vi "VGA_Loop.vi"   [LabVIEW 2019, in "VGA.lvlib"]
doc: "Contains the Loop to handle the VGA Output. It constantly outputs the FrameBuffer Memory. Update the FrameBuffer or change Initial-value of the Memory to display something."
uses:
  VGA.lvlib
  data.ctl
  <vilib>/Platform/TimedLoop/XDataNode/timing_clust.ctl
  <vilib>/Platform/TimedLoop/XDataNode/nitl_modes.ctl
  <vilib>/Platform/TimedLoop/XDataNode/wakeup.ctl
  <vilib>/rvi/Emulation/niFpgaSctlEmulationGetInTimedLoop.vi
  <vilib>/rvi/Emulation/niFpgaEmulationReportErrorSimple.vi
  <vilib>/rvi/Emulation/niFpgaGetClockAttributes.vi
  <vilib>/rvi/Emulation/niFpgaCriticalErrorInLSC.vi
  <vilib>/rvi/eio/common/nirviEmuTemplateMethod_errors.vi
  <vilib>/platform/TimedLoop/XDataNode/XDataNode.xnode
  <vilib>/eio/EIONode/EIONode.xnode
  <vilib>/Platform/TimedLoop/XDataNode/XDNodeRunTimeDep.lvlib
types:
  T1 = typedef "VGA.lvlib/data.ctl" = cluster{"x_frontporch":u8, "x_syncpulse":u8, "x_backporch":u8, "y_frontporch":u8, "y_syncpulse":u8, "y_backporch":u8, "DrawPixel?":bool, "x_tickcount":u16, "y_tickcount":u16, "x_Index":i16, "y_Index":i16}
  T2 = typedef "XDNodeRunTimeDep.lvlib/timing_clust.ctl" = cluster{"Expected End [f-1]":u64, "Actual End [f-1]":u64, "Finished Late? [f-1]":bool, "Expected End [i-1]":u64, "Actual End [i-1]":u64, "Finished Late? [i-1]":bool, "Expected Start [i]":u64, "Actual Start [i]":u64, "Expected Start [f]":u64, "Actual Start [f]":u64, "Source Name":string, "Structure Name":string, "Period":i64, "Deadline":i64, "Offset":i64, "Start":i64, "Priority":i32, "Timeout":i32, "Mode":T3, "Wakeup Reason":T4, "Error":errorcluster, "Source Type":string, "Secondary Source Type":string, "Global End Time":u64, "Global Start Time":u64, "Frame Duration":u64, "Iteration Duration":u64, "Assigned CPU":i32, "I/O Scan Engine Mode":u32}
  T3 = typedef "XDNodeRunTimeDep.lvlib/nitl_modes.ctl" = enum32{"No Change", "Process missed periods, maintain original phase", "Discard missed periods, maintain original phase", "Process missed periods, ignore original phase", "Discard missed periods, ignore original phase"}
  T4 = typedef "XDNodeRunTimeDep.lvlib/wakeup.ctl" = enum32{"Normal", "Aborted", "Asynchronous wakeup", "Timing source error", "Timed loop error", "Timeout"}
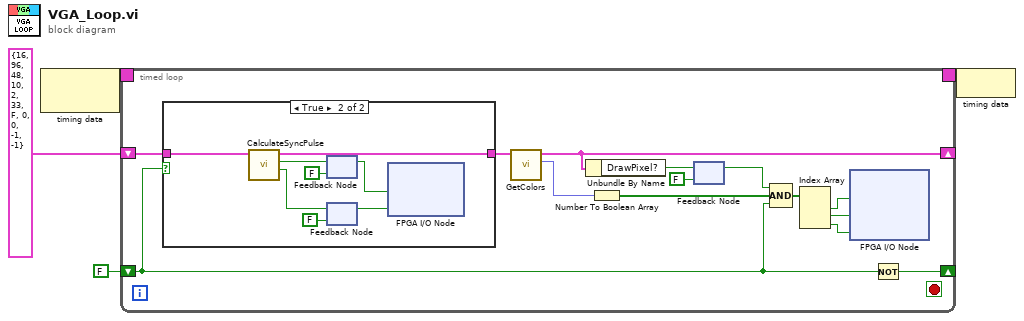
[diagram p0: block diagram]
diagram:
  n1 = node-c288() -> (w4:T2)  [unwired: 1 in]
  n2 = timed-loop {
    timing: w4 -> [_]
    timing-out: [_] -> w3
    shift-right: [w11] -> _
    shift-left: T1 {"x_frontporch"=16, "x_syncpulse"=96, "x_backporch"=48, "y_frontporch"=10, "y_syncpulse"=2, "y_backporch"=33, "DrawPixel?"=FALSE, "x_tickcount"=0, "y_tickcount"=0, "x_Index"=-1, "y_Index"=-1} ("VGA_data") -> [w18]
    shift-right: [w14] -> _
    shift-left: FALSE -> [w12]
    stop <- _ stop-if-true
    n3 = case shown="True" w12 {
      tunnel: w18 -> [w19 w27]
      tunnel: [w19 w26] -> w17
      frame False {
      }
      frame True {
        n4 = call "CalculateSyncPulse.vi"("VGA_data"=w27) -> ("vSync"=w25:bool, "hSync"=w24:bool, "VGA_data 2"=w26:T1)  [unwired: 8 in]
        n5 = feedback-in #1(w24) -> ()
        n6 = feedback #1(FALSE ("hSync")) -> (w23:bool)
        n7 = feedback-in #2(w25) -> ()
        n8 = feedback #2(FALSE ("vSync")) -> (w22:bool)
        n9 = xnode "FPGA I/O Node"("hSync"=w23, "vSync"=w22) -> ()  [unwired: 2 in, 2 out]
      }
    }
    n10 = call "GetColors.vi"("VGA_data"=w17) -> ("Colors"=w16:fxp<+,3,3>, "VGA_data 2"=w11:T1)  [unwired: 9 in]
    n11 = Unbundle By Name(w11) -> ("DrawPixel?"=w10:bool)
    n12 = Number To Boolean Array(number=w16) -> (Boolean array=w15:bool[])
    n13 = feedback #3(FALSE ("DrawPixel?")) -> (w6:bool)
    n14 = feedback-in #3(w10) -> ()
    n15 = Compound Arithmetic op=AND(w6, w15, w12) -> (w13:bool[])
    n16 = Index Array(array=w13) -> (element #1=w9:bool, element #2=w8:bool, element #3=w7:bool)  [unwired: 3 in]
    n17 = xnode "FPGA I/O Node"("RED"=w9, "GREEN"=w8, "BLUE"=w7) -> ()  [unwired: 3 in, 3 out]
    n18 = Not(x=w12) -> (.not. x?=w14:bool)
  }
  n19 = node-c288(w3) -> ()
